vi "ExampleRestartableWriter.vi"() -> ()   [LabVIEW 2011]
uses:
  0x2 Typedefs/RIO-OCU update controls.ctl
  2-Think/2 Typedefs/generalized sensor status.ctl
  2-Think/2 Typedefs/indicator LED.ctl
  2-Think/2 Typedefs/generalized actuator status.ctl
  2-Think/2 Typedefs/Which Boat.ctl
  2-Think/2 Typedefs/robot velocity.ctl
  2-Think/2 Typedefs/UTM Location.ctl
  2-Think/2 Typedefs/heading.ctl
  2-Think/2 Typedefs/rate of turn.ctl
  2-Think/2 Typedefs/pitch and roll.ctl
  2-Think/2 Typedefs/apparent wind.ctl
  2-Think/2 Typedefs/apparent wind speed.ctl
  2-Think/2 Typedefs/apparent wind direction.ctl
  2-Think/2 Typedefs/Velocity.ctl
  2-Think/2 Typedefs/absolute wind direction.ctl
  2-Think/2 Typedefs/absolute wind speed.ctl
  2-Think/2 Typedefs/absolute water current vector.ctl
  2-Think/2 Typedefs/rudder angle.ctl
  2-Think/2 Typedefs/sail setpt.ctl
  0x2 Typedefs/manual override.ctl
  2-Think/2 Typedefs/setpoints to boat.ctl
  0x2 Typedefs/Current Waypoint.ctl
  2-Think/2 Typedefs/Goodness Fns Indicator.ctl
  2-Think/2 Typedefs/UTM Circle.ctl
  2-Think/2 Globals/2 Global.vi
  Writer/NetworkStreamWriter.lvclass
panel:
  out "Connected?":bool
  in  "Monitored Items from RIO":T1 {"Absolute Wind"."East" format="%#_5g"; "Robot Pitch/Roll"."Roll" format="%05.1f"; "Robot Pitch/Roll"."Pitch" format="%05.1f"; "Robot\nRate of Turn" format="%05.1f"; "Robot\nHeading" format="%05.1f"; "Robot UTM Location"."North" format="%#_10f"; "Robot UTM Location"."East" format="%#_8f"}
  out "Current iteration":i32
  in  "stop":bool
  # "How Am I?"
  # "Where Am I?"
  # "Path Planning"
  # "From Planning Functions"
  # "(this is not a cluster because subitems\nare generated in parallel code)"
  # "What's Around Me?"
  # "As Measured"
  # "As Measured"
  # "Loop Rates"
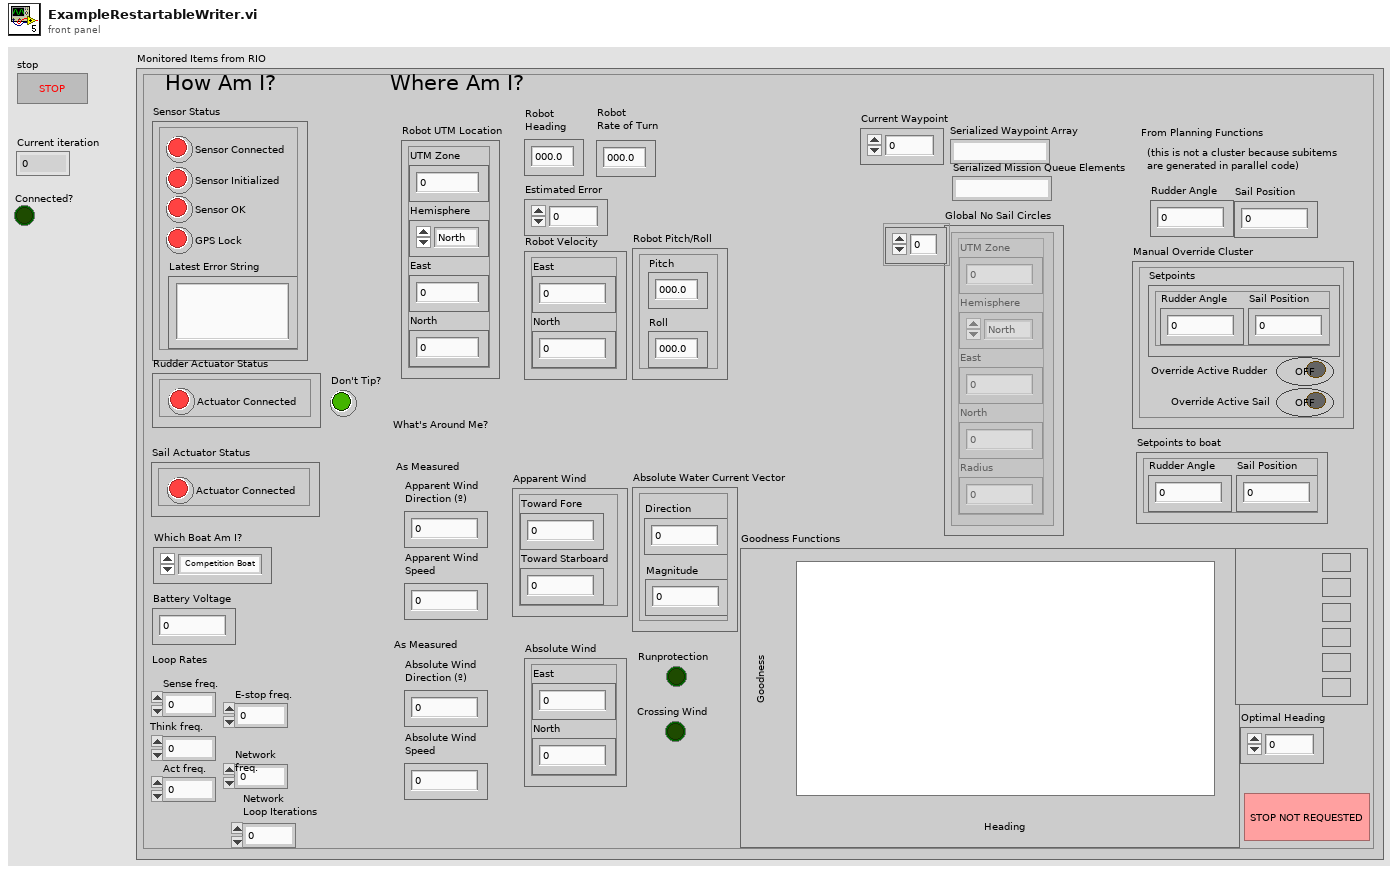
[diagram p1: front panel]
types:
  T1 = typedef "RIO-OCU update controls.ctl" = cluster{"Sensor Status":T2, "Battery Voltage":dbl, "Rudder Actuator Status":T4, "Sail Actuator Status":T4, "Which Boat Am I?":T5, "Robot Velocity":T6, "Robot UTM Location":T7, "Robot\nHeading ":T8, "Robot\nRate of Turn":T9, "Robot Pitch/Roll":T10, "Apparent Wind":T11, "Apparent Wind\nSpeed":T12, "Apparent Wind\nDirection (º)":T13, "Absolute Wind":T14, "Absolute Wind\nDirection (º)":T15, "Absolute Wind\nSpeed":T16, "Absolute Water Current Vector":T17, "Rudder Angle":T18, "Sail Position":T19, "Manual Override Cluster":T20, "Setpoints to boat":T21, "Current Waypoint":T22, "Think freq.":dbl, "Sense freq.":dbl, "Act freq.":dbl, "E-stop freq.":dbl, "Network \nfreq.":dbl, "Network \nLoop Iterations":i64, "E-Stop":bool, "Serialized Waypoint Array":string, "Serialized Mission Queue Elements":string, "Goodness Functions":T23, "Global No Sail Circles":T24[], "Runprotection":bool, "Optimal Heading":dbl, "Crossing Wind":bool, "Estimated Error":dbl, "Don't Tip?":bool}
  T2 = typedef "generalized sensor status.ctl" = cluster{"Sensor Connected":T3, "Sensor Initialized":T3, "Sensor OK":T3, "Latest Error String":string, "GPS Lock":T3}
  T3 = typedef "indicator LED.ctl" = bool
  T4 = typedef "generalized actuator status.ctl" = cluster{"Actuator Connected":T3}
  T5 = typedef "Which Boat.ctl" = enum16{"Competition Boat", "Small RC", "Simulation"}
  T6 = typedef "robot velocity.ctl" = cluster{"East":dbl, "North":dbl}
  T7 = typedef "UTM Location.ctl" = cluster{"UTM Zone":dbl, "Hemisphere":enum16{"North", "South"}, "East":dbl, "North":dbl}
  T8 = typedef "heading.ctl" = dbl
  T9 = typedef "rate of turn.ctl" = dbl
  T10 = typedef "pitch and roll.ctl" = cluster{"Pitch":dbl, "Roll":dbl}
  T11 = typedef "apparent wind.ctl" = cluster{"Toward Fore":dbl, "Toward Starboard":dbl}
  T12 = typedef "apparent wind speed.ctl" = dbl
  T13 = typedef "apparent wind direction.ctl" = dbl
  T14 = typedef "Velocity.ctl" = cluster{"East":dbl, "North":dbl}
  T15 = typedef "absolute wind direction.ctl" = dbl
  T16 = typedef "absolute wind speed.ctl" = dbl
  T17 = typedef "absolute water current vector.ctl" = cluster{"Direction":T13, "Magnitude":T13}
  T18 = typedef "rudder angle.ctl" = dbl
  T19 = typedef "sail setpt.ctl" = dbl
  T20 = typedef "manual override.ctl" = cluster{"Override Active Rudder":bool, "Setpoints":T21, "Override Active Sail":bool}
  T21 = typedef "setpoints to boat.ctl" = cluster{"Sail Position":T19, "Rudder Angle":T18}
  T22 = typedef "Current Waypoint.ctl" = i32
  T23 = typedef "Goodness Fns Indicator.ctl" = cluster{dbl, dbl, dbl[][]}
  T24 = typedef "UTM Circle.ctl" = cluster{"UTM Zone":dbl, "Hemisphere":enum16{"North", "South"}, "East":dbl, "North":dbl, "Radius":dbl}
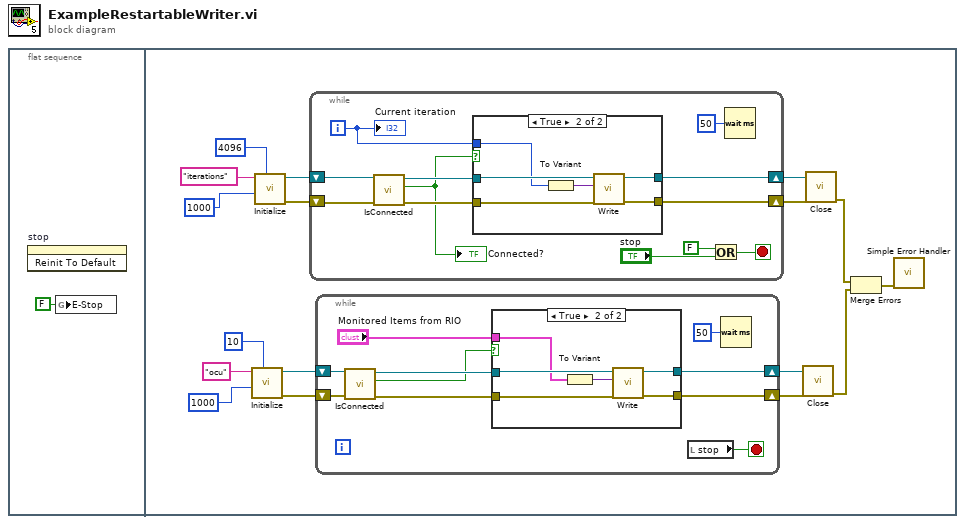
[diagram p0: block diagram]
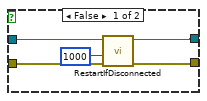
[diagram p2: hidden frame]
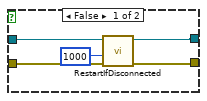
[diagram p3: hidden frame]
diagram:
  n1 = flat-sequence {
    frame #0 {
      n2 = invoke on="stop" class="Bool (strict)" method="Reinit To Default"() -> ()  [unwired: 3 in, 3 out]
      n3 = global write "2 Global.vi" "E-Stop"(FALSE ("E-Stop")) -> ()
    }
    frame #1 {
      n4 = call "Initialize.vi"("writer buffer size"=10, "connection timeout"=1000, "writer name"="ocu") -> ("error out"=w10:errorcluster, "NetworkStreamWriter out"=w9:refnum<class "NetworkStreamWriter.lvclass">)  [unwired: 6 in, 1 out]
      n5 = call "Initialize.vi"("writer buffer size"=4096, "connection timeout"=1000, "writer name"="iterations") -> ("error out"=w17:errorcluster, "NetworkStreamWriter out"=w18:refnum<class "NetworkStreamWriter.lvclass">)  [unwired: 6 in, 1 out]
      n6 = while {
        shift-right: [w40] -> w14
        shift-left: w17 -> [w44]
        shift-right: [w41] -> w15
        shift-left: w18 -> [w45]
        i -> [w43]
        stop <- w49 stop-if-true
        n7 = call "IsConnected.vi"("error in (no error)"=w44, "NetworkStreamWriter in"=w45) -> ("error out"=w46:errorcluster, "Connected?"=w42:bool, "NetworkStreamWriter out"=w47:refnum<class "NetworkStreamWriter.lvclass">)  [unwired: 7 in]
        "Connected?" <- w42
        n8 = case shown="True" w42 {
          tunnel: w47 -> [w55 w61]
          tunnel: w46 -> [w54 w58]
          tunnel: w43 -> [_ w60]
          tunnel: [w53 w59] -> w41
          tunnel: [w52 w57] -> w40
          frame False {
            n9 = call "RestartIfDisconnected.vi"("error in (no error)"=w54, "connection timeout"=1000, "NetworkStreamWriter in"=w55) -> ("error out"=w52:errorcluster, "NetworkStreamWriter out"=w53:refnum<class "NetworkStreamWriter.lvclass">)  [unwired: 7 in]
          }
          frame True {
            n10 = To Variant(anything=w60) -> (Variant=w62:variant)
            n11 = call "Write.vi"("error in (no error)"=w58, "element"=w62, "NetworkStreamWriter in"=w61) -> ("error out"=w57:errorcluster, "NetworkStreamWriter out"=w59:refnum<class "NetworkStreamWriter.lvclass">)  [unwired: 6 in, 1 out]
          }
        }
        n12 = Or(x=FALSE, y="stop") -> (x .or. y?=w49:bool)
        n13 = Wait (ms)(milliseconds to wait=u32 50) -> ()  [unwired: 1 out]
        "Current iteration" <- w43
      }
      n14 = while {
        shift-right: [w19] -> w13
        shift-left: w10 -> [w25]
        shift-right: [w20] -> w12
        shift-left: w9 -> [w26]
        stop <- w27 stop-if-true
        n15 = call "IsConnected.vi"("error in (no error)"=w25, "NetworkStreamWriter in"=w26) -> ("error out"=w22:errorcluster, "Connected?"=w23:bool, "NetworkStreamWriter out"=w24:refnum<class "NetworkStreamWriter.lvclass">)  [unwired: 7 in]
        n16 = case shown="True" w23 {
          tunnel: w24 -> [w32 w38]
          tunnel: w22 -> [w31 w35]
          tunnel: "Monitored Items from RIO" -> [_ w37]
          tunnel: [w30 w36] -> w20
          tunnel: [w29 w34] -> w19
          frame False {
            n17 = call "RestartIfDisconnected.vi"("error in (no error)"=w31, "connection timeout"=1000, "NetworkStreamWriter in"=w32) -> ("error out"=w29:errorcluster, "NetworkStreamWriter out"=w30:refnum<class "NetworkStreamWriter.lvclass">)  [unwired: 7 in]
          }
          frame True {
            n18 = To Variant(anything=w37) -> (Variant=w39:variant)
            n19 = call "Write.vi"("error in (no error)"=w35, "element"=w39, "NetworkStreamWriter in"=w38) -> ("error out"=w34:errorcluster, "NetworkStreamWriter out"=w36:refnum<class "NetworkStreamWriter.lvclass">)  [unwired: 6 in, 1 out]
          }
        }
        n20 = local read "stop"() -> (w27:bool)
        n21 = Wait (ms)(milliseconds to wait=u32 50) -> ()  [unwired: 1 out]
      }
      n22 = call "Close.vi"("error in (no error)"=w13, "NetworkStreamWriter in"=w12) -> ("error out"=w7:errorcluster)  [unwired: 8 in, 1 out]
      n23 = call "Close.vi"("error in (no error)"=w14, "NetworkStreamWriter in"=w15) -> ("error out"=w8:errorcluster)  [unwired: 8 in, 1 out]
      n24 = Merge Errors(w8, w7) -> (w6:errorcluster)
      n25 = call <vilib>:"Simple Error Handler.vi"("error in (no error)"=w6) -> ()  [unwired: 4 in, 5 out]
    }
  }
